vi "Motor_firmware.vi"(8 "error in (no error)":errorcluster, 10 "Main Code":string="# https://github.com/tinkertechtrove/pico-pi-playing/blob/main/pio-steppers/test_motor4.py\n# Motor:  https://www.amazon.com/gp/product/B094YQBYB9/ref=ppx_yo_dt_b_search_asin_title?ie=UTF8&psc=1\n#Wiring: Black to A+ Green to A- Red to B+ Blue to B-\n# A+, B+, A-, B- = so Black, Red, Green, Blue with the values below\n\nfrom machine import Pin\nfrom rp2 import PIO, StateMachine, asm_pio\nfrom time import sleep\nimport sys\n\nrelay = Pin(3, Pin.OUT)  # was 27 for the cytron\nrelay.off()\n\ndef pulse():\n    relay.on()\n    sleep(0.1)\n    relay.off()\n\n@asm_pio(set_init=(PIO.OUT_LOW,) * 4, out_init=(PIO.OUT_LOW,) * 4, out_shiftdir=PIO.SHIFT_RIGHT, in_shiftdir=PIO.SHIFT_LEFT)\n        \ndef prog():\n    pull() \n    mov(x, osr)\n    pull() \n    mov(y, osr)\n    \n    jmp(not_x, \"end\") \n    \n    label(\"loop\")  \n    jmp(not_osre, \"step\") \n    mov(osr, y)  \n    label(\"step\") \n    out(pins, 4) [31]\n    jmp(x_dec,\"loop\")\n    label(\"end\")\n    irq(rel(0))  #fire interrupt that you are done\n\nsm = StateMachine(0, prog, freq=3200, set_base=Pin(8), out_base=Pin(8))\nCCW = [0b0001,0b0010,0b0100,0b1000,0b0001,0b0010,0b0100,0b1000]  #stepper patterns\nCW =  CCW.copy() #stepper patterns\nCW.reverse()\n\nsteps = 0\nrunning = False\n\ndef turn(sm, goal = 200, CW_dir = True):  # callback when done\n    global steps, running\n    \n    sleep(1)  # pause\n    CW_dir = goal < steps\n    data = CW if CW_dir else CCW\n    pulse = abs(goal - steps)\n    a = 0\n    for i,byte in enumerate(data):\n        a += byte << i*4\n    print(\"Going to send {0:b}\".format(a))\n    sm.put(pulse)\n    sm.put(a)\n    running = True\n    steps = (steps - pulse) if CW_dir else (steps + pulse)\n    \ndef flip(sm):\n    global running\n    running = False\n\ndef waiting():\n    while running:\n        sleep(0.5)\n\nsm.irq(flip)\n", 11 "VISA Refnum in":refnum<visa-resource-name>) -> (0 "error out":errorcluster, 2 "reply":string)   [LabVIEW 2022 SP3]
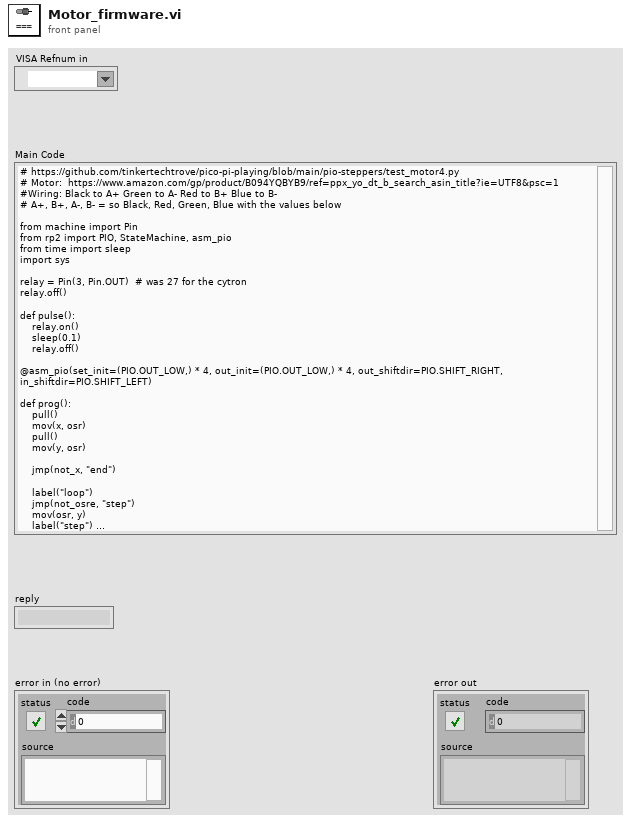
[diagram p1: front panel]
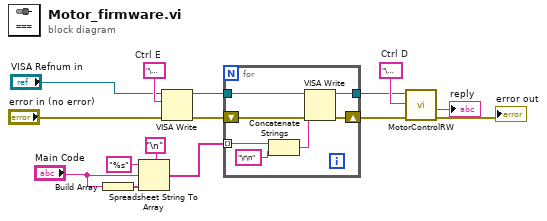
[diagram p0: block diagram]
diagram:
  w14 = "\u0004"  # Ctrl D
  w7 = "\u0005"  # Ctrl E
  n1 = Build Array("Main Code") -> (w3:string[])
  n2 = Spreadsheet String To Array(delimiter (Tab)="\n", format string="%s", spreadsheet string="Main Code", array type (2D Dbl)=w3) -> (array=w2:string[])
  n3 = VISA Write(VISA resource name="VISA Refnum in", write buffer=w7, error in (no error)="error in (no error)") -> (VISA resource name out=w8:refnum<visa-resource-name>, error out=w9:errorcluster)  [unwired: 1 out]
  n4 = for {
    tunnel: w2 -> [w22] mode=indexing
    tunnel: w8 -> [w19]
    tunnel: [w18] -> w13
    shift-right: [w16] -> w12
    shift-left: w9 -> [w17]
    n5 = Concatenate Strings(w22, "\r\n" ("delimiter (Tab)")) -> (w20:string)
    n6 = VISA Write(VISA resource name=w19, write buffer=w20, error in (no error)=w17) -> (VISA resource name out=w18:refnum<visa-resource-name>, error out=w16:errorcluster)  [unwired: 1 out]
  }
  n7 = call "MotorControlRW.vi"("error in (no error)"=w12, "payload"=w14, "VISA in"=w13) -> ("error out"=→"error out":errorcluster, "reply"=→"reply":string)  [unwired: 4 in, 3 out]
